vi "ClickReleaseMouseLeft.vi"(11 "click/release":bool) -> ()   [LabVIEW 2013]
uses:
  User32.dll
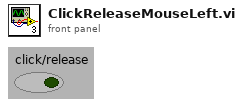
[diagram p1: front panel]
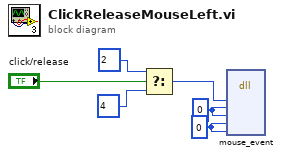
[diagram p0: block diagram]
diagram:
  w3 = 0 ("dwExtraInfo")
  w2 = u32 0 ("dwExtraInfo")
  n1 = Select(t=2, s="click/release", f=4) -> (s? t:f=w1:i32)
  n2 = dll-call lib="user32.dll" fn="mouse_event" label="Click"("dwFlags"=w1, "dx"=w3, "dy"=w3, "dwData"=w2, "dwExtraInfo"=w2) -> ()  [unwired: 9 in, 2 out]
